vi "PXDAC4800_SetPowerUpDefaultsXD48.vi"(0 "Handle":u32) -> (1 "Status":i32, 2 "Handle out":u32)   [LabVIEW 2016]
uses:
  PXDAC4800.dll
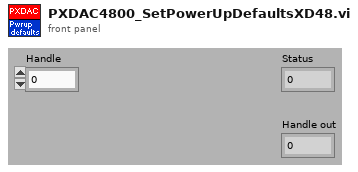
[diagram p1: front panel]
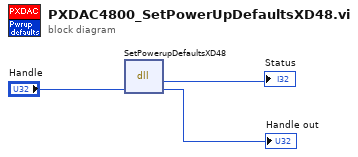
[diagram p0: block diagram]
diagram:
  n1 = dll-call lib="PXDAC4800.dll" fn="SetPowerupDefaultsXD48"("Handle"="Handle") -> (→"Status":i32, "Handle"=→"Handle out":u32)  [unwired: 3 in, 2 out]
